vi "一体站流程自动启动.vi"(11 "参数":T1) -> ()   [LabVIEW 2016, in "PLC.lvlib"]
uses:
  PLC.lvlib
  <vilib>/ptbypt/NI_PtbyPt.lvlib
panel:
  out "s? t:f":enum16{"初始化", "采配水启动", "仪器操作", "反冲洗", "结束"}(ring)
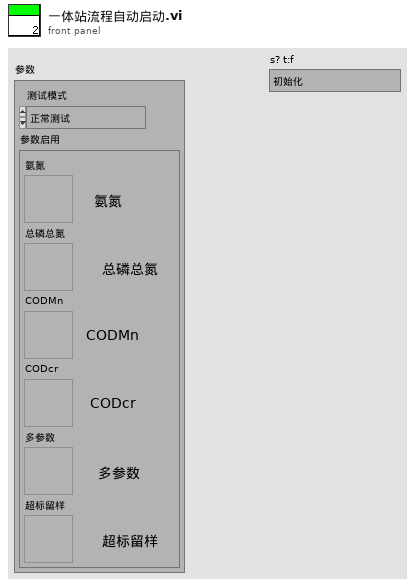
[diagram p1: front panel]
types:
  T1 = cluster{"测试模式":enum16{"正常测试", "集成干预"}, "参数启用":cluster{"氨氮":bool, "总磷总氮":bool, "CODMn":bool, "CODcr":bool, "多参数":bool, "超标留样":bool}}
  T2 = cluster{"命令":string, cluster{"starting address":u16, "holding register value":u16}}
  T3 = enum16{"启动测量", "标样核查", "零点核查", "跨度核查", "空白测试", "平行样测试", "加标回收", "空白校准", "标样校准", "初始化（清洗）", "停止测试", "仪器重启", "校时", "模式设置", "测量间隔设置"}
  T4 = cluster{"时间标识":timestamp, "设备":string, "日志信息":string, "流程参数":string}
  T5 = cluster{"测量模式":enum16{"水样测量", "标样核查", "零点核查", "跨度核查", "空白测试", "加标回收", "平行样", "校零", "校标"}}
  T6 = cluster{"时间标识":timestamp, "设备":string, "日志信息":string}
  T7 = enum16{"空闲", "水样测试", "标样核查", "零点核查", "跨度核查", "空白测试", "平行样测试", "加标回收", "空白校准", "标样校准", "初始化（清洗）"}
  T8 = enum32{"Bad", "Idle", "Run top level", "Running"}
  T9 = cluster{"R0":i16, "R1":i16, "R2":i16, "R3":i16, "R4":i16, "R5":i16, "R6":i16, "R7":i16, "R8":i16, "R9":i16, "R10":i16, "R11":i16, "R12":i16, "R13":i16, "R14":i16, "R15":i16, "R16":i16, "R17":i16, "R18":i16, "R19":i16, "R20":i16, "R21":i16, "R22":i16, "R23":i16, "R24":i16, "R25":i16, "R26":i16, "R27":i16, "R28":i16, "R29":i16, "R30":i16, "R31":i16, "R32":i16, "R33":i16, "R34":i16, "R35":i16, "R36":i16, "R37":i16, "R38":i16, "R39":i16, "R40":i16, "R41":i16, "R42":i16, "R43":i16, "R44":i16, "R45":i16, "R46":i16, "R47":i16, "R48":i16, "R49":i16, "R50":i16, "R51":i16, "R52":i16, "R53":i16, "R54":i16, "R55":i16, "R56":i16}
  T10 = cluster{"R100":i16, "R101":i16, "R102":i16, "R103":i16, "R104":i16, "R105":i16, "R106":i16, "R107":i16, "R108":i16, "R109":i16, "R110":i16, "R111":i16, "R112":i16, "R113":i16, "R114":i16, "R115":i16, "R116":i16, "R117":i16, "R118":i16, "R119":i16, "R120":i16, "R121":i16, "R122":i16, "R123":i16, "R124":i16}
  T11 = cluster{"氨氮":bool, "总磷总氮":bool, "CODmn":bool, "CODCr":bool, "多参数":bool, "超标留样":bool}
  T12 = cluster{"因子编码":u32, "单位":u16, "标样参考值":sgl, "水样数据时间":timestamp, "水样实测值":sgl, "水样数据标识":string, "标样数据时间":timestamp, "标样实测值":sgl, "标样数据标识":string, "空白数据时间":timestamp, "空白实测值":sgl, "空白数据标识":string, "零点核查数据时间":timestamp, "零点核查实测值":sgl, "零点核查数据标识":string, "跨度核查数据时间":timestamp, "跨度核查实测值":sgl, "跨度核查数据标识":string, "加标回收数据时间":timestamp, "加标回收实测值":sgl, "加标回收数据标识":string, "平行样数据时间":timestamp, "平行样实测值":sgl, "平行样数据标识":string, "F0":sgl, "F1":sgl, "F2":sgl, "F3":sgl, "F4":sgl, "F5":sgl, "F6":sgl, "F7":sgl, "温度":sgl, "湿度":sgl, "X值":sgl, "fidrange":u16}
  T13 = cluster{"COD浓度（mg/L)":dbl, "水样启动时间":timestamp, "加标回收启动时间":timestamp, "CODMn工作状态":enum16{"空闲", "水样测试", "标样核查", "零点核查", "跨度核查", "空白测试", "平行样测试", "加标回收", "空白校准", "标样校准", "初始化（清洗）"}, "多列列表框":i32}
  T14 = cluster{"因子编码":u32, "单位":u16, "标样参考值":sgl, "水样数据时间":timestamp, "水样实测值":sgl, "水样数据标识":string, "标样数据时间":timestamp, "标样实测值":sgl, "标样数据标识":string, "空白数据时间":timestamp, "空白实测值":sgl, "空白数据标识":string, "零点核查数据时间":timestamp, "零点核查实测值":sgl, "零点核查数据标识":string, "跨度核查数据时间":timestamp, "跨度核查实测值":sgl, "跨度核查数据标识":string, "加标回收数据时间":timestamp, "加标回收实测值":sgl, "加标回收数据标识":string, "平行样数据时间":timestamp, "平行样实测值":sgl, "平行样数据标识":string}
  T15 = cluster{"氨氮":bool, "总磷总氮":bool, "CODMn":bool, "CODcr":bool, "多参数":bool, "超标留样":bool}
  T16 = cluster{"时间标识":timestamp, "参数":string, "数据类型":string, "集成干预测试浓度值":dbl, "集成干预前测试时间":timestamp, "集成干预前测试浓度值":dbl}
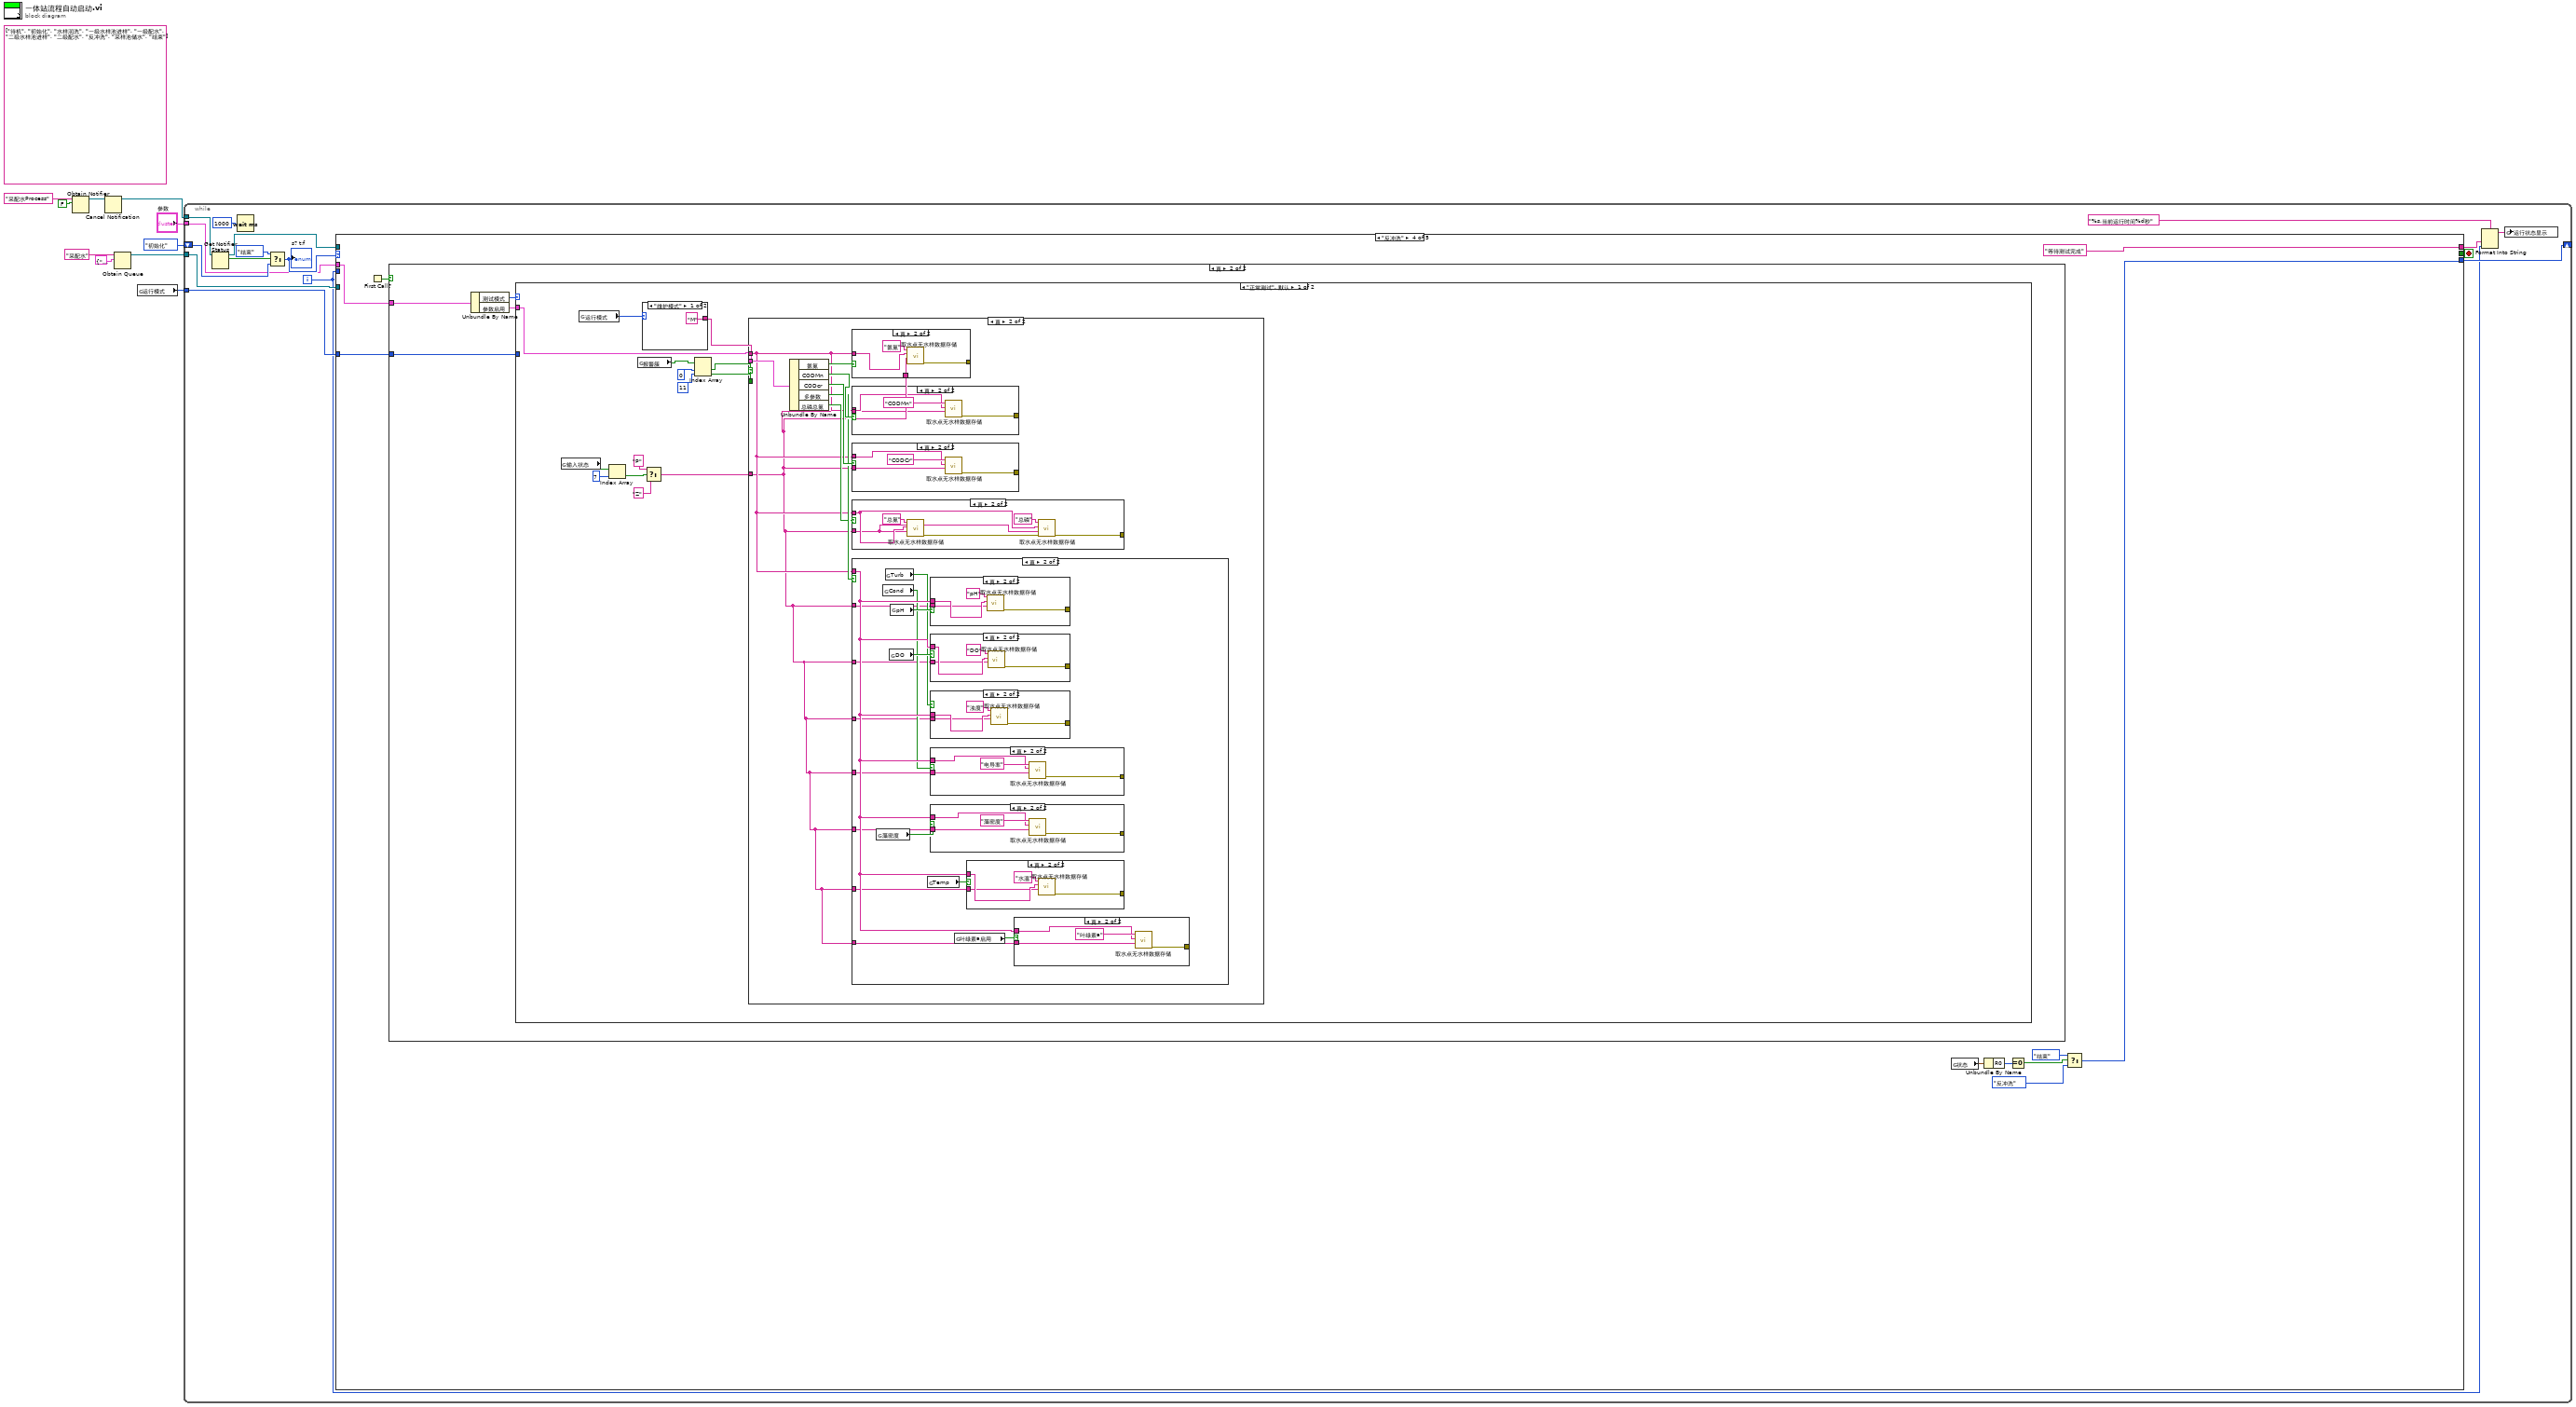
[diagram p0: block diagram]
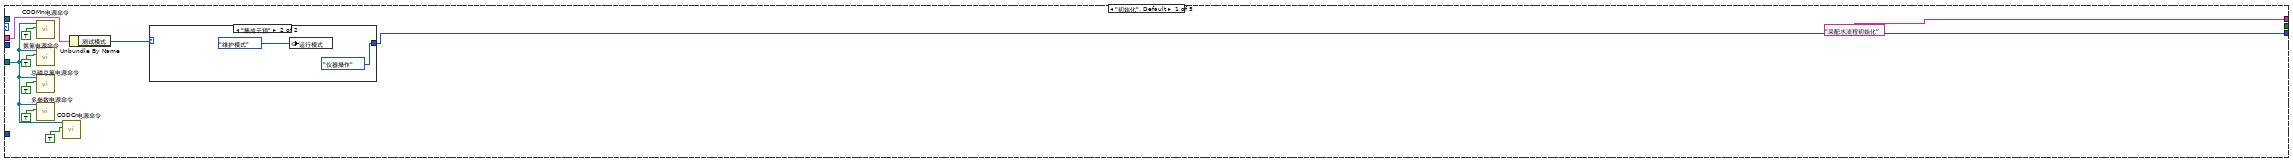
[diagram p2: hidden frame]
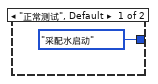
[diagram p3: hidden frame]
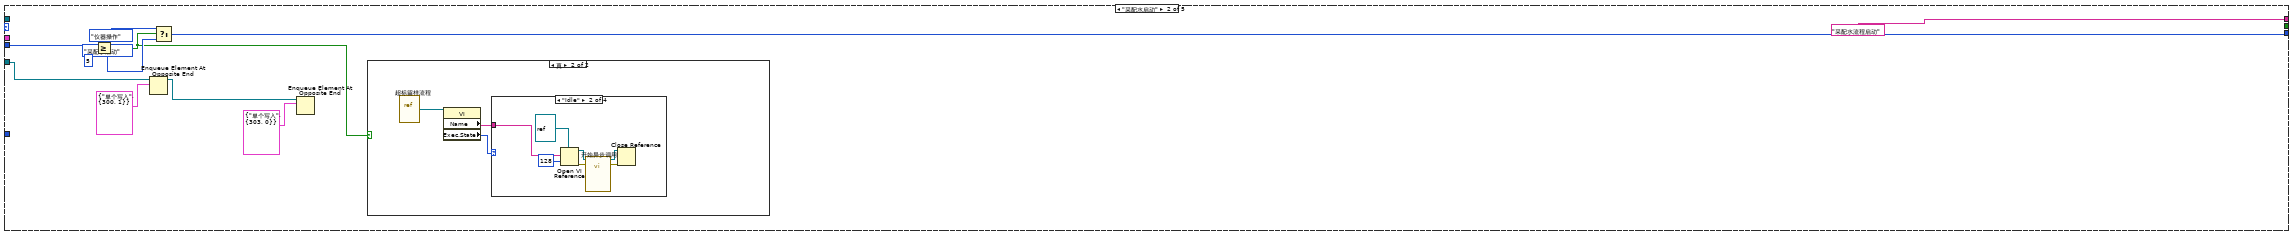
[diagram p4: hidden frame]
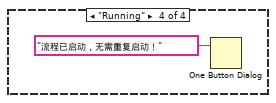
[diagram p8: hidden frame]
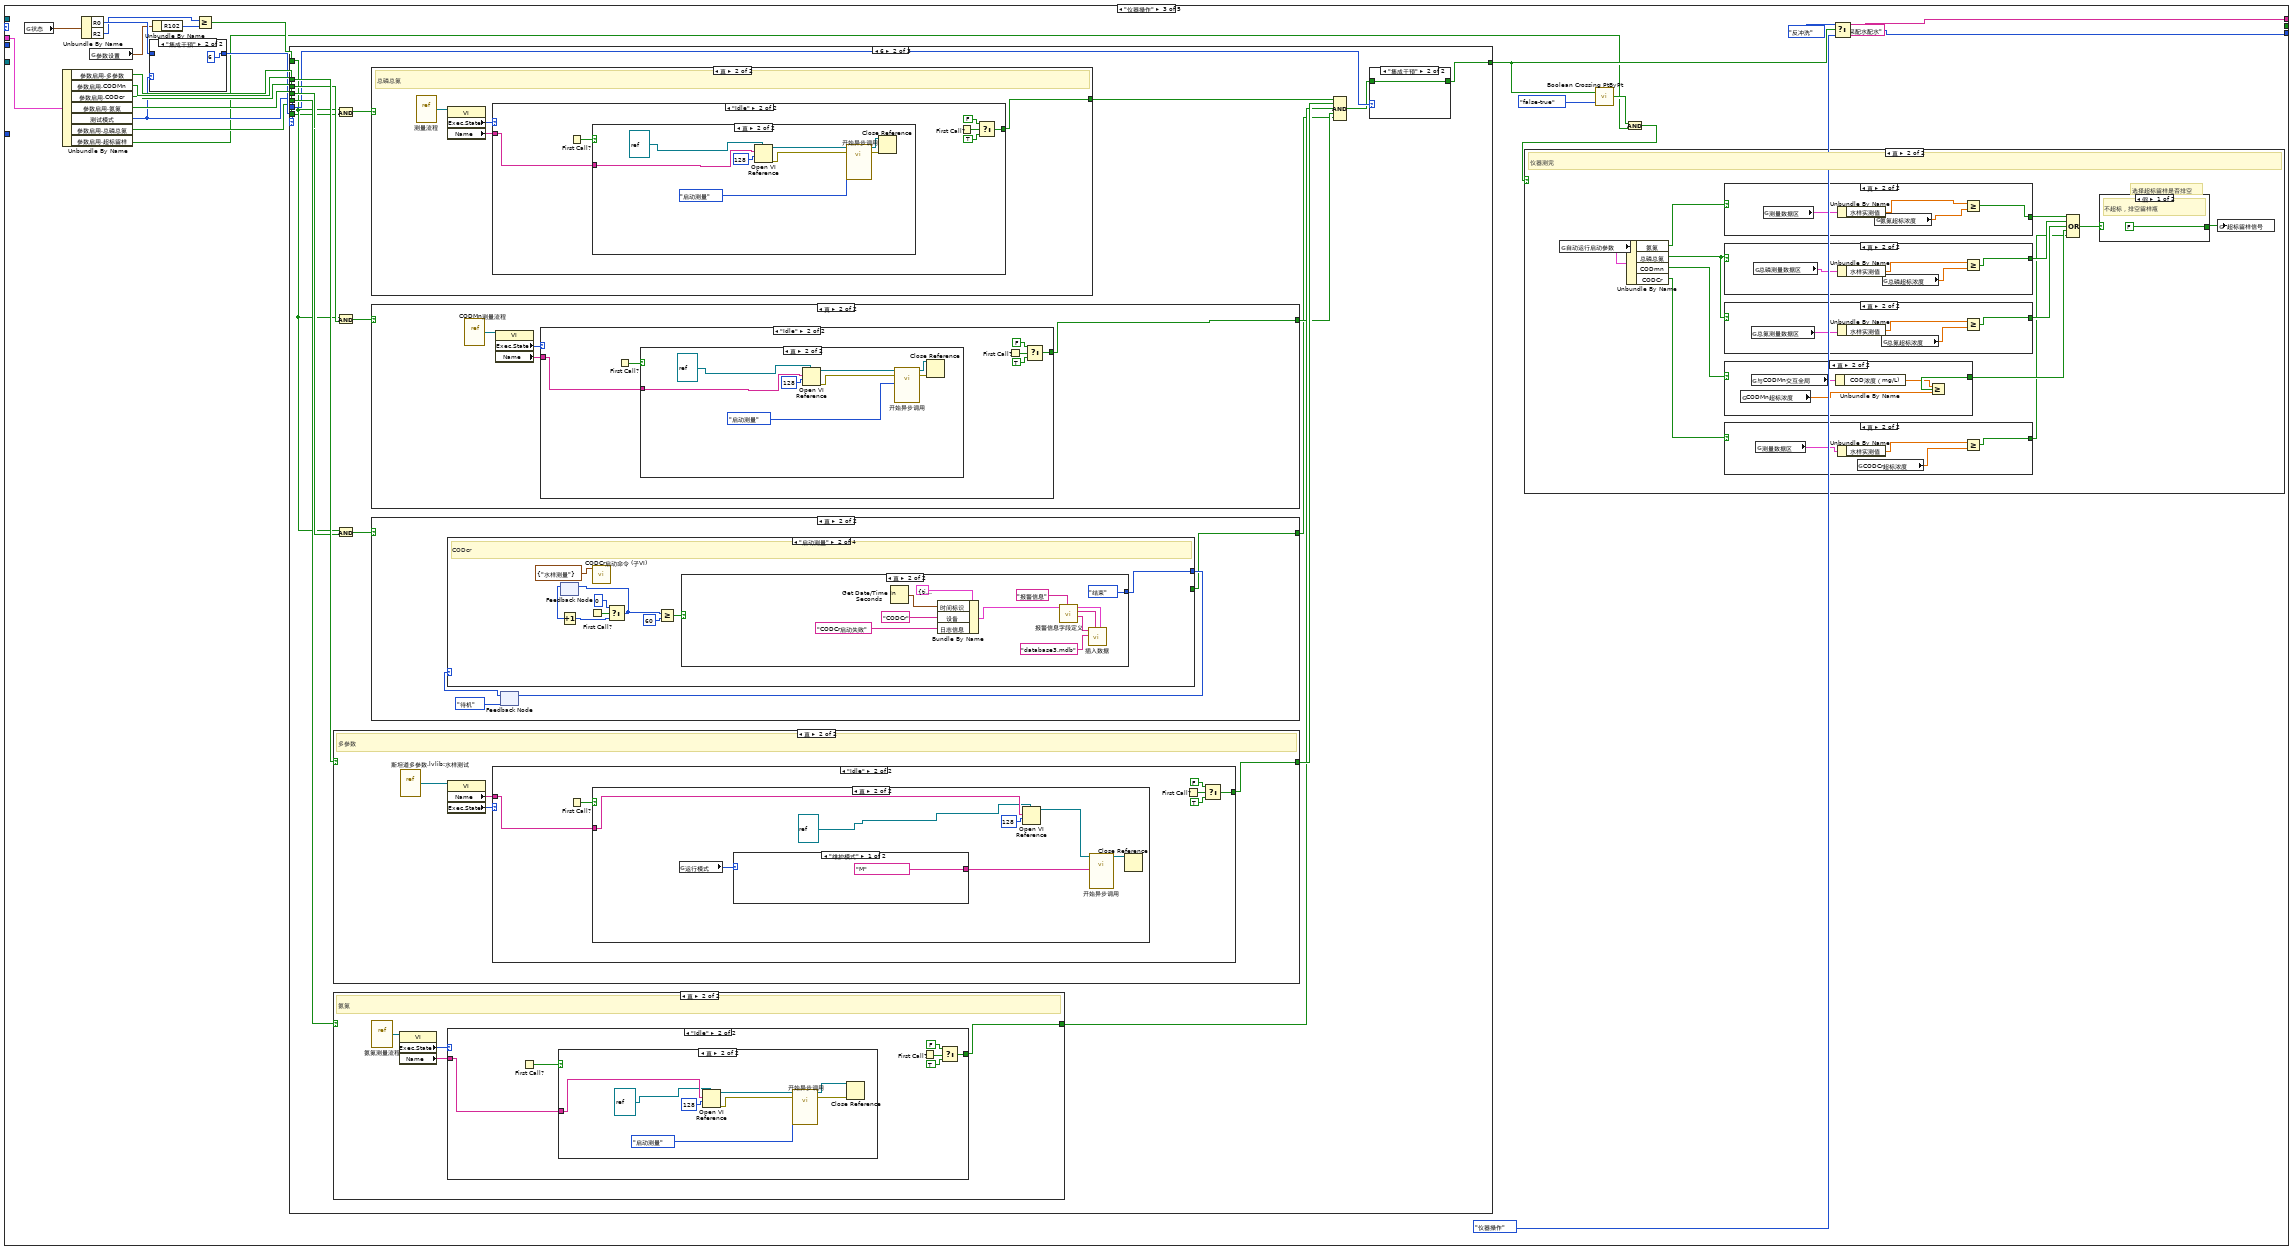
[diagram p9: hidden frame]
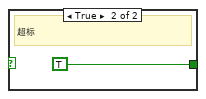
[diagram p11: hidden frame]
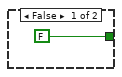
[diagram p12: hidden frame]
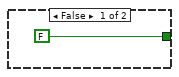
[diagram p13: hidden frame]
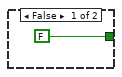
[diagram p14: hidden frame]
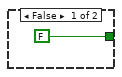
[diagram p15: hidden frame]
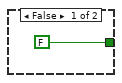
[diagram p16: hidden frame]
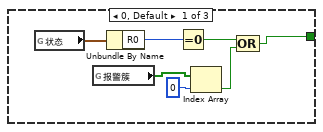
[diagram p18: hidden frame]
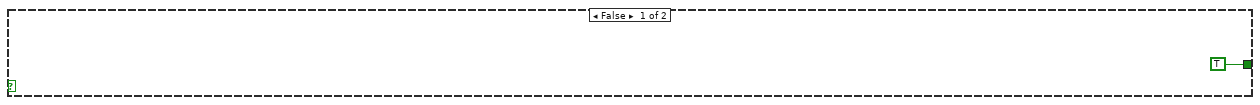
[diagram p19: hidden frame]
diagram:
  (unwired) string[][] [["待机"], ["初始化"], ["水样润洗"], ["一级水样池进样"], ["一级配水"], ["二级水样池进样"], ["二级配水"], ["反冲洗"], ["采样池储水"], ["结束"]] ("项名")
  n1 = Obtain Notifier(name (unnamed)="采配水Process" ("名称（未命名）"), notification data type=FALSE) -> (notifier out=w4:refnum<notifier>)  [unwired: 2 in, 2 out]
  n2 = Cancel Notification(0:w4) -> (8:w3:refnum<notifier>)  [unwired: 1 in, 2 out]
  n3 = Obtain Queue(name (unnamed)="采配水" ("名称（未命名）"), element data type=cluster{"命令":string, "数据":variant} {"命令"="", "数据"=variant}) -> (queue out=w7:refnum<queue>)  [unwired: 3 in, 2 out]
  n4 = global read "系统设置全局变量.vi" "运行模式"() -> (w1:enum16{"维护模式", "常规模式", "应急模式", "质控模式"})
  n5 = while {
    shift-right: [w23] -> _
    shift-left: enum16{"初始化", "采配水启动", "仪器操作", "反冲洗", "结束"}."初始化" ("枚举") -> [w19]
    tunnel: w7 -> [w26]
    tunnel: w3 -> [w22]
    tunnel: "参数" -> [w13]
    tunnel: w1 -> [w12]
    i -> [w11]
    stop <- w25 stop-if-true
    n6 = Get Notifier Status(notifier=w22) -> (notifier out=w14:refnum<notifier>, current notification=w21:bool)  [unwired: 1 in, 3 out]
    n7 = Wait (ms)(milliseconds to wait=u32 1000 ("等待时间（毫秒）")) -> ()  [unwired: 1 out]
    n8 = Select(t=enum16{"初始化", "采配水启动", "仪器操作", "反冲洗", "结束"}."结束" ("枚举"), s=w21, f=w19) -> (s? t:f=w18:enum16{"初始化", "采配水启动", "仪器操作", "反冲洗", "结束"})
    "s? t:f" <- w18
    n9 = case shown="\"反冲洗\"" w18 {
      tunnel: w26 -> [w31 w50 _ _ w476]
      tunnel: [_ _ _ _ TRUE] -> w25
      tunnel: [w30 w43 w80 w285 enum16{"初始化", "采配水启动", "仪器操作", "反冲洗", "结束"}."结束" ("枚举")] -> w23
      tunnel: ["采配水流程初始化" "采配水流程启动" "采配水配水" "等待测试完成" "采配水结束"] -> w15
      tunnel: w14 -> [_ _ _ _ w477]
      tunnel: w13 -> [w28 _ w82 w284 w473]
      tunnel: w12 -> [_ _ _ w281 w472]
      tunnel: w11 -> [_ w48 _ _ _]
      frame "初始化", Default {
        n10 = call "CODMn电源命令.vi"("通电/断电"=TRUE, "队列"=w31) -> ()  [unwired: 9 in, 1 out]
        n11 = call "氨氮电源命令.vi"("通电/断电"=TRUE, "队列"=w31) -> ()  [unwired: 9 in, 1 out]
        n12 = call "总磷总氮电源命令.vi"("通电/断电"=TRUE, "队列"=w31) -> ()  [unwired: 9 in, 1 out]
        n13 = call "多参数电源命令.vi"("通电/断电"=TRUE, "队列"=w31) -> ()  [unwired: 9 in, 1 out]
        n14 = call "CODCr电源命令.vi"("通电/断电"=TRUE, "队列"=w31) -> ()  [unwired: 9 in, 1 out]
        n15 = Unbundle By Name(w28) -> ("测试模式"=w27:enum16{"正常测试", "集成干预"})
        n16 = case shown="\"集成干预\"" w27 {
          tunnel: [enum16{"初始化", "采配水启动", "仪器操作", "反冲洗", "结束"}."采配水启动" ("枚举") enum16{"初始化", "采配水启动", "仪器操作", "反冲洗", "结束"}."仪器操作" ("枚举")] -> w30
          frame "正常测试", Default {
          }
          frame "集成干预" {
            n17 = global write "系统设置全局变量.vi" "运行模式"(enum16{"维护模式", "常规模式", "应急模式", "质控模式"}."维护模式" ("运行模式")) -> ()
          }
        }
      }
      frame "采配水启动" {
        n18 = Greater Or Equal?(x=w48, y=5) -> (x >= y?=w40:bool)
        n19 = Enqueue Element At Opposite End(queue=w50, element=T2 {"命令"="单个写入", {"starting address"=300, "holding register value"=1}} ("元素")) -> (queue out=w41:refnum<queue>)  [unwired: 2 in, 2 out]
        n20 = Select(t=enum16{"初始化", "采配水启动", "仪器操作", "反冲洗", "结束"}."仪器操作" ("枚举"), s=w40, f=enum16{"初始化", "采配水启动", "仪器操作", "反冲洗", "结束"}."采配水启动" ("枚举")) -> (s? t:f=w43:enum16{"初始化", "采配水启动", "仪器操作", "反冲洗", "结束"})
        n21 = Enqueue Element At Opposite End(queue=w41, element=T2 {"命令"="单个写入", {"starting address"=303, "holding register value"=0}} ("元素")) -> ()  [unwired: 2 in, 3 out]
        n22 = case shown="真" w40 {
          frame False {
          }
          frame True {
            n23 = vi-ref "超标留样流程.vi"() -> (w53:refnum<vi>)
            n24 = property class="VI"(reference=w53) -> ("Name"=w52:string, "Exec.State"=w51:T8)  [unwired: 1 in, 2 out]
            n25 = case shown="\"Idle\"" w51 {
              tunnel: w52 -> [_ w56 _ _]
              frame "Bad", Default {
              }
              frame "Idle" {
                n26 = Open VI Reference(type specifier VI Refnum (for type only)=refnum<vi> refnum ("类型说明符VI引用句柄（仅用于类型）"), vi path=w56, options=128 ("选项")) -> (vi reference=w60:refnum<vi>, error out=w55:errorcluster)  [unwired: 3 in]
                n27 = call-by-ref "开始异步调用"(reference=w60, error in=w55) -> (reference out=w59:refnum<vi>, error out=w54:errorcluster)  [unwired: 12 in]
                n28 = Close Reference(reference=w59, error in (no error)=w54) -> ()  [unwired: 1 out]
              }
              frame "Run top level" {
              }
              frame "Running" {
                n29 = One Button Dialog(message="流程已启动，无需重复启动！" ("消息")) -> ()  [unwired: 1 in, 1 out]
              }
            }
          }
        }
      }
      frame "仪器操作" {
        n30 = global read "采配水全局变量.vi" "状态"() -> (w84:T9)
        n31 = Unbundle By Name(w82) -> ("参数启用.多参数"=w78:bool, "参数启用.CODMn"=w77:bool, "参数启用.CODcr"=w76:bool, "参数启用.氨氮"=w75:bool, "测试模式"=w68:enum16{"正常测试", "集成干预"}, "参数启用.总磷总氮"=w67:bool, "参数启用.超标留样"=w62:bool)
        n32 = Unbundle By Name(w84) -> ("R0"=w74:i16, "R2"=w69:i16)
        n33 = global read "采配水全局变量.vi" "参数设置"() -> (w71:T10)
        n34 = case shown="\"集成干预\"" w68 {
          tunnel: w74 -> [w124 _]
          tunnel: [w124 i16 6 ("R0")] -> w73
          frame "正常测试", Default {
          }
          frame "集成干预" {
          }
        }
        n35 = Unbundle By Name(w71) -> ("R102"=w72:i16)
        n36 = Greater Or Equal?(x=w69, y=w72) -> (x >= y?=w70:bool)
        n37 = case shown="6" w73 {
          tunnel: [w127 w137 TRUE] -> w63
          tunnel: w78 -> [_ w149 _]
          tunnel: w77 -> [_ w148 _]
          tunnel: w76 -> [_ w145 _]
          tunnel: w75 -> [_ w144 _]
          tunnel: w70 -> [_ w136 _]
          tunnel: w68 -> [_ w139 _]
          tunnel: w67 -> [_ w135 _]
          frame 0, Default {
            n38 = global read "采配水全局变量.vi" "状态"() -> (w130:T9)
            n39 = global read "采配水全局变量.vi" "报警簇"() -> (w131:bool[])
            n40 = Unbundle By Name(w130) -> ("R0"=w129:i16)
            n41 = Equal To 0?(x=w129) -> (x = 0?=w132:bool)
            n42 = Index Array(array=w131, index=0 ("索引")) -> (element=w126:bool)
            n43 = Compound Arithmetic op=OR ("复合运算")(w132, w126) -> (w127:bool)
          }
          frame 6 {
            n44 = case shown="真" w149 {
              tunnel: [TRUE ("t") w261] -> w143
              frame False {
              }
              frame True {
                # "多参数"
                n45 = vi-ref "斯坦道多参数.lvlib:水样测试.vi"() -> (w263:refnum<vi>)
                n46 = property class="VI"(reference=w263) -> ("Name"=w262:string, "Exec.State"=w264:T8)  [unwired: 1 in, 2 out]
                n47 = case shown="\"Idle\"" w264 {
                  tunnel: w262 -> [_ w270]
                  tunnel: [_ w265] -> w261
                  frame "Bad", Default {
                  }
                  frame "Idle" {
                    n48 = First Call?() -> (First Call?: T/F=w269:bool)
                    n49 = case shown="真" w269 {
                      tunnel: w270 -> [_ w276]
                      frame False {
                      }
                      frame True {
                        n50 = global read "系统设置全局变量.vi" "运行模式"() -> (w273:enum16{"维护模式", "常规模式", "应急模式", "质控模式"})
                        n51 = case shown="\"维护模式\"" w273 {
                          tunnel: ["M" ("数据标记表") "N" ("数据标记表")] -> w272
                          frame "维护模式" {
                          }
                          frame "常规模式", Default {
                          }
                        }
                        n52 = Open VI Reference(type specifier VI Refnum (for type only)=refnum<vi> refnum, vi path=w276, options=128 ("选项")) -> (vi reference=w275:refnum<vi>)  [unwired: 3 in, 1 out]
                        n53 = call-by-ref "开始异步调用"(reference=w275, "数据标记表"=w272) -> (reference out=w274:refnum<vi>)  [unwired: 12 in, 1 out]
                        n54 = Close Reference(reference=w274) -> ()  [unwired: 1 in, 1 out]
                      }
                    }
                    n55 = First Call?() -> (First Call?: T/F=w268:bool)
                    n56 = Select(t=FALSE, s=w268, f=TRUE) -> (s? t:f=w265:bool)
                  }
                }
              }
            }
            n57 = case "条件结构" shown="真" w144 {
              tunnel: [TRUE ("t") w171] -> w142
              frame False {
              }
              frame True {
                # "氨氮"
                n58 = vi-ref "氨氮测量流程.vi"() -> (w174:refnum<vi>)
                n59 = property class="VI"(reference=w174) -> ("Exec.State"=w173:T8, "Name"=w172:string)  [unwired: 1 in, 2 out]
                n60 = case shown="\"Idle\"" w173 {
                  tunnel: w172 -> [_ w180]
                  tunnel: [_ w175] -> w171
                  frame "Bad", Default {
                  }
                  frame "Idle" {
                    n61 = First Call?() -> (First Call?: T/F=w179:bool)
                    n62 = case shown="真" w179 {
                      tunnel: w180 -> [_ w185]
                      frame False {
                      }
                      frame True {
                        n63 = Open VI Reference(type specifier VI Refnum (for type only)=refnum<vi> refnum, vi path=w185, options=128 ("选项")) -> (vi reference=w183:refnum<vi>, error out=w186:errorcluster)  [unwired: 3 in]
                        n64 = call-by-ref "开始异步调用"(reference=w183, error in=w186, "控制命令"=T3."启动测量") -> (reference out=w187:refnum<vi>, error out=w188:errorcluster)  [unwired: 11 in]
                        n65 = Close Reference(reference=w187, error in (no error)=w188) -> ()  [unwired: 1 out]
                      }
                    }
                    n66 = First Call?() -> (First Call?: T/F=w178:bool)
                    n67 = Select(t=FALSE, s=w178, f=TRUE) -> (s? t:f=w175:bool)
                  }
                }
              }
            }
            n68 = And(x=w136, y=w135) -> (x .and. y?=w134:bool)
            n69 = And(x=w136, y=w148) -> (x .and. y?=w147:bool)
            n70 = And(x=w136, y=w145) -> (x .and. y?=w146:bool)
            n71 = case "条件结构" shown="真" w134 {
              tunnel: [TRUE ("t") w151] -> w133
              frame False {
              }
              frame True {
                # "总磷总氮"
                n72 = vi-ref "测量流程.vi"() -> (w154:refnum<vi>)
                n73 = property class="VI"(reference=w154) -> ("Exec.State"=w153:T8, "Name"=w152:string)  [unwired: 1 in, 2 out]
                n74 = case shown="\"Idle\"" w153 {
                  tunnel: w152 -> [_ w160]
                  tunnel: [_ w155] -> w151
                  frame "Bad", Default {
                  }
                  frame "Idle" {
                    n75 = First Call?() -> (First Call?: T/F=w159:bool)
                    n76 = case shown="真" w159 {
                      tunnel: w160 -> [_ w165]
                      frame False {
                      }
                      frame True {
                        n77 = Open VI Reference(type specifier VI Refnum (for type only)=refnum<vi> refnum, vi path=w165, options=128 ("选项")) -> (vi reference=w163:refnum<vi>, error out=w166:errorcluster)  [unwired: 3 in]
                        n78 = call-by-ref "开始异步调用"(reference=w163, error in=w166, "控制命令"=T3."启动测量") -> (reference out=w167:refnum<vi>, error out=w168:errorcluster)  [unwired: 11 in]
                        n79 = Close Reference(reference=w167, error in (no error)=w168) -> ()  [unwired: 1 out]
                      }
                    }
                    n80 = First Call?() -> (First Call?: T/F=w158:bool)
                    n81 = Select(t=FALSE, s=w158, f=TRUE) -> (s? t:f=w155:bool)
                  }
                }
              }
            }
            n82 = case shown="真" w147 {
              tunnel: [TRUE w242] -> w141
              frame False {
              }
              frame True {
                n83 = vi-ref "CODMn测量流程.vi"() -> (w243:refnum<vi>)
                n84 = property class="VI"(reference=w243) -> ("Exec.State"=w244:T8, "Name"=w245:string)  [unwired: 1 in, 2 out]
                n85 = case shown="\"Idle\"" w244 {
                  tunnel: w245 -> [_ w251]
                  tunnel: [_ w246] -> w242
                  frame "Bad", Default {
                  }
                  frame "Idle" {
                    n86 = First Call?() -> (First Call?: T/F=w250:bool)
                    n87 = case shown="真" w250 {
                      tunnel: w251 -> [_ w256]
                      frame False {
                      }
                      frame True {
                        n88 = Open VI Reference(type specifier VI Refnum (for type only)=refnum<vi> refnum, vi path=w256, options=128 ("选项")) -> (vi reference=w254:refnum<vi>, error out=w257:errorcluster)  [unwired: 3 in]
                        n89 = call-by-ref "开始异步调用"(reference=w254, error in=w257, "控制命令"=T3."启动测量") -> (reference out=w258:refnum<vi>, error out=w259:errorcluster)  [unwired: 11 in]
                        n90 = Close Reference(reference=w258, error in (no error)=w259) -> ()  [unwired: 1 out]
                      }
                    }
                    n91 = First Call?() -> (First Call?: T/F=w249:bool)
                    n92 = Select(t=FALSE, s=w249, f=TRUE) -> (s? t:f=w246:bool)
                  }
                }
              }
            }
            n93 = case shown="真" w146 {
              tunnel: [TRUE w190] -> w140
              frame False {
              }
              frame True {
                n94 = feedback #1(enum16{"待机", "启动测量", "测量中", "结束"}."待机") -> (w192:enum16{"待机", "启动测量", "测量中", "结束"})
                n95 = case shown="\"启动测量\"" w192 {
                  tunnel: [enum16{"待机", "启动测量", "测量中", "结束"}."启动测量" w208 w228 enum16{"待机", "启动测量", "测量中", "结束"}."结束"] -> w191
                  tunnel: [_ _ _ TRUE] -> w190
                  frame "待机", Default {
                    n96 = Get Date/Time In Seconds() -> (seconds since 1Jan1904=w198:timestamp)
                    n97 = Bundle By Name(cluster=T4 {"时间标识"=timestamp(0 s since 1904-01-01), "设备"="", "日志信息"="", "流程参数"=""} ("data in"), "时间标识"=w198, "设备"="CODCr", "日志信息"="-->>CODCr启动") -> (w194:T4)
                    n98 = call "总磷总氮操作日志.vi"("data in"=w194) -> ()  [unwired: 11 in]
                  }
                  frame "启动测量" {
                    # "CODcr"
                    n99 = feedback #2() -> (w204:i32)  [unwired: 1 in]
                    n100 = Increment(x=w204) -> (x+1=w205:i32)
                    n101 = First Call?() -> (First Call?: T/F=w203:bool)
                    n102 = call "CODCr启动命令 (子VI).vi"("启动测量模式"=T5 {"测量模式"=enum."水样测量"}) -> ()  [unwired: 11 in]
                    n103 = Select(t=0, s=w203, f=w205) -> (s? t:f=w206:i32)
                    n104 = feedback-in #2(w206) -> ()
                    n105 = Greater Or Equal?(x=w206, y=60) -> (x >= y?=w201:bool)
                    n106 = case shown="真" w201 {
                      tunnel: [w209 enum16{"待机", "启动测量", "测量中", "结束"}."结束"] -> w208
                      frame False {
                        n107 = global read "CODcr全局变量.vi" "工作状态"() -> (w210:T7)
                        n108 = Not Equal To 0?(x=w210) -> (x != 0?=w211:bool)
                        n109 = Select(t=enum16{"待机", "启动测量", "测量中", "结束"}."测量中", s=w211, f=enum16{"待机", "启动测量", "测量中", "结束"}."启动测量") -> (s? t:f=w209:enum16{"待机", "启动测量", "测量中", "结束"})
                      }
                      frame True {
                        n110 = Get Date/Time In Seconds() -> (seconds since 1Jan1904=w220:timestamp)
                        n111 = Bundle By Name(cluster=T6 {"时间标识"=timestamp(0 s since 1904-01-01), "设备"="", "日志信息"=""} ("data in"), "时间标识"=w220, "设备"="CODCr", "日志信息"="CODCr启动失败") -> (w214:T6)
                        n112 = call "报警信息字段定义.vi"("table输入"="报警信息", "data in"=w214) -> ("table输出"=w217:string, "columns"=w218:string[], "data out"=w219:T6)  [unwired: 7 in]
                        n113 = call "插入数据.vi"("data"=w219, "columns"=w218, "database"="database3.mdb", "table"=w217) -> ()  [unwired: 7 in, 1 out]
                      }
                    }
                  }
                  frame "测量中" {
                    n114 = global read "CODcr全局变量.vi" "工作状态"() -> (w227:T7)
                    n115 = Equal?(x=w227, y=T7."空闲" ("工作状态")) -> (x = y?=w226:bool)
                    n116 = case shown="假" w226 {
                      tunnel: [w229 enum16{"待机", "启动测量", "测量中", "结束"}."结束"] -> w228
                      frame False {
                        n117 = flat-sequence {
                          tunnel: [enum16{"待机", "启动测量", "测量中", "结束"}."测量中"] -> w229
                          frame #0 {
                            n118 = Wait (ms)(milliseconds to wait=u32 1000 ("等待时间（毫秒）")) -> ()  [unwired: 1 out]
                          }
                          frame #1 {
                          }
                        }
                      }
                      frame True {
                      }
                    }
                  }
                  frame "结束" {
                    n119 = First Call?() -> (First Call?: T/F=w233:bool)
                    n120 = case shown="真" w233 {
                      frame False {
                      }
                      frame True {
                        n121 = Get Date/Time In Seconds() -> (seconds since 1Jan1904=w240:timestamp)
                        n122 = Bundle By Name(cluster=T4 {"时间标识"=timestamp(0 s since 1904-01-01), "设备"="", "日志信息"="", "流程参数"=""} ("data in"), "时间标识"=w240, "设备"="CODCr", "日志信息"="-->>CODCr停止") -> (w236:T4)
                        n123 = call "总磷总氮操作日志.vi"("data in"=w236) -> ()  [unwired: 11 in]
                      }
                    }
                  }
                }
                n124 = feedback-in #1(w191) -> ()
              }
            }
            n125 = Compound Arithmetic op=AND ("复合运算")(w133, w143, w142, w141, w140) -> (w138:bool)
            n126 = case shown="\"集成干预\"" w139 {
              tunnel: w138 -> [_ w169]
              tunnel: [_ w169] -> w137
              frame "正常测试", Default {
              }
              frame "集成干预" {
              }
            }
          }
          frame 7..9 {
          }
        }
        n127 = call <vilib>:"Boolean Crossing PtByPt.vi"("direction"=enum16{"either", "false-true", "true-false"}."false-true", "input"=w63) -> ("crossing"=w65:bool)  [unwired: 1 in]
        n128 = And(x=w65, y=w62) -> (x .and. y?=w64:bool)
        n129 = case shown="真" w64 {
          frame False {
          }
          frame True {
            # "选择超标留样是否排空"
            # "仪器测完"
            n130 = global read "系统设置全局变量.vi" "自动运行启动参数"() -> (w89:T11)
            n131 = Unbundle By Name(w89) -> ("氨氮"=w88:bool, "总磷总氮"=w87:bool, "CODmn"=w86:bool, "CODCr"=w85:bool)
            n132 = case shown="真" w88 {
              tunnel: [FALSE w122] -> w96
              frame False {
              }
              frame True {
                n133 = global read "VAR氨氮全局变量.vi" "测量数据区"() -> (w121:T12)
                n134 = Unbundle By Name(w121) -> ("水样实测值"=w123:sgl)
                n135 = global read "外部交互全局.vi" "氨氮超标浓度"() -> (w120:dbl)
                n136 = Greater Or Equal?(x=w123, y=w120) -> (x >= y?=w122:bool)
              }
            }
            n137 = case shown="真" w87 {
              tunnel: [FALSE w118] -> w95
              frame False {
              }
              frame True {
                n138 = global read "VAR总磷总氮全局变量.vi" "总磷测量数据区"() -> (w115:T12)
                n139 = Unbundle By Name(w115) -> ("水样实测值"=w117:sgl)
                n140 = global read "外部交互全局.vi" "总磷超标浓度"() -> (w116:dbl)
                n141 = Greater Or Equal?(x=w117, y=w116) -> (x >= y?=w118:bool)
              }
            }
            n142 = case shown="真" w87 {
              tunnel: [FALSE w113] -> w94
              frame False {
              }
              frame True {
                n143 = global read "VAR总磷总氮全局变量.vi" "总氮测量数据区"() -> (w110:T12)
                n144 = Unbundle By Name(w110) -> ("水样实测值"=w112:sgl)
                n145 = global read "外部交互全局.vi" "总氮超标浓度"() -> (w111:dbl)
                n146 = Greater Or Equal?(x=w112, y=w111) -> (x >= y?=w113:bool)
              }
            }
            n147 = case shown="真" w86 {
              tunnel: [FALSE w108] -> w93
              frame False {
              }
              frame True {
                n148 = global read "外部交互全局.vi" "CODMn超标浓度"() -> (w107:dbl)
                n149 = global read "modbus slave全局.vi" "与CODMn交互全局"() -> (w106:T13)
                n150 = Unbundle By Name(w106) -> ("COD浓度（mg/L)"=w105:dbl)
                n151 = Greater Or Equal?(x=w105, y=w107) -> (x >= y?=w108:bool)
              }
            }
            n152 = case shown="真" w85 {
              tunnel: [FALSE w103] -> w92
              frame False {
              }
              frame True {
                n153 = global read "CODcr全局变量.vi" "测量数据区"() -> (w100:T14)
                n154 = Unbundle By Name(w100) -> ("水样实测值"=w102:sgl)
                n155 = global read "外部交互全局.vi" "CODCr超标浓度"() -> (w101:dbl)
                n156 = Greater Or Equal?(x=w102, y=w101) -> (x >= y?=w103:bool)
              }
            }
            n157 = Compound Arithmetic op=OR ("复合运算")(w96, w95, w94, w93, w92) -> (w91:bool)
            n158 = case shown="假" w91 {
              tunnel: [FALSE ("超标留样信号") TRUE ("超标留样信号")] -> w90
              frame False {
                # "不超标，排空留样瓶"
              }
              frame True {
                # "超标"
              }
            }
            n159 = global write "外部交互全局.vi" "超标留样信号"(w90) -> ()
          }
        }
        n160 = Select(t=enum16{"初始化", "采配水启动", "仪器操作", "反冲洗", "结束"}."反冲洗" ("枚举"), s=w63, f=enum16{"初始化", "采配水启动", "仪器操作", "反冲洗", "结束"}."仪器操作" ("枚举")) -> (s? t:f=w80:enum16{"初始化", "采配水启动", "仪器操作", "反冲洗", "结束"})
      }
      frame "反冲洗" {
        n161 = First Call?() -> (First Call?: T/F=w282:bool)
        n162 = case shown="真" w282 {
          tunnel: w284 -> [_ w294]
          tunnel: w281 -> [_ w291]
          frame False {
          }
          frame True {
            n163 = Unbundle By Name(w294) -> ("测试模式"=w293:enum16{"正常测试", "集成干预"}, "参数启用"=w292:T15)
            n164 = case shown="\"正常测试\", 默认" w293 {
              tunnel: w292 -> [w303 w396]
              tunnel: w291 -> [_ w390]
              frame "正常测试", Default {
                n165 = global read "采配水全局变量.vi" "输入状态"() -> (w300:bool[])
                n166 = global read "系统设置全局变量.vi" "运行模式"() -> (w301:enum16{"维护模式", "常规模式", "应急模式", "质控模式"})
                n167 = Index Array(array=w300, index=7 ("索引")) -> (element=w298:bool)
                n168 = global read "采配水全局变量.vi" "报警簇"() -> (w308:bool[])
                n169 = case shown="\"维护模式\"" w301 {
                  tunnel: ["M" ("table") "N" ("table")] -> w302
                  frame "维护模式" {
                  }
                  frame "常规模式", Default {
                  }
                }
                n170 = Select(t="P" ("数据标识"), s=w298, f="Z" ("数据标识")) -> (s? t:f=w295:string)
                n171 = Index Array(array=w308, index #1=0 ("索引"), index #2=11 ("索引")) -> (element #1=w305:bool, element #2=w304:bool)
                n172 = case shown="真" w305 {
                  tunnel: w304 -> [w314 _]
                  tunnel: w303 -> [w313 w328]
                  tunnel: w302 -> [w311 w322]
                  tunnel: w295 -> [_ w321]
                  frame False {
                    n173 = Unbundle By Name(w313) -> ("氨氮"=w312:bool)
                    n174 = case shown="真" w314 {
                      tunnel: w312 -> [_ w316]
                      tunnel: w311 -> [_ w315]
                      frame False {
                      }
                      frame True {
                        n175 = case shown="真" w316 {
                          tunnel: w315 -> [_ w317]
                          tunnel: [_ w318] -> _
                          frame False {
                          }
                          frame True {
                            n176 = call "取水点无水样数据存储.vi"("数据标识"="lw", "数据类型"=w317, "table"="氨氮") -> ("error out"=w318:errorcluster)  [unwired: 8 in]
                          }
                        }
                      }
                    }
                  }
                  frame True {
                    n177 = Unbundle By Name(w328) -> ("氨氮"=w327:bool, "CODMn"=w326:bool, "CODcr"=w325:bool, "多参数"=w324:bool, "总磷总氮"=w323:bool)
                    n178 = case shown="真" w327 {
                      tunnel: w322 -> [_ w387]
                      tunnel: [_ w388] -> _
                      tunnel: w321 -> [_ w386]
                      frame False {
                      }
                      frame True {
                        n179 = call "取水点无水样数据存储.vi"("数据标识"=w386, "数据类型"=w387, "table"="氨氮") -> ("error out"=w388:errorcluster)  [unwired: 8 in]
                      }
                    }
                    n180 = case shown="真" w326 {
                      tunnel: w322 -> [_ w384]
                      tunnel: [_ w383] -> _
                      tunnel: w321 -> [_ w382]
                      frame False {
                      }
                      frame True {
                        n181 = call "取水点无水样数据存储.vi"("数据标识"=w382, "数据类型"=w384, "table"="CODMn") -> ("error out"=w383:errorcluster)  [unwired: 8 in]
                      }
                    }
                    n182 = case shown="真" w325 {
                      tunnel: w322 -> [_ w380]
                      tunnel: [_ w379] -> _
                      tunnel: w321 -> [_ w378]
                      frame False {
                      }
                      frame True {
                        n183 = call "取水点无水样数据存储.vi"("数据标识"=w378, "数据类型"=w380, "table"="CODCr") -> ("error out"=w379:errorcluster)  [unwired: 8 in]
                      }
                    }
                    n184 = case shown="真" w323 {
                      tunnel: w322 -> [_ w331]
                      tunnel: [_ w330] -> _
                      tunnel: w321 -> [_ w329]
                      frame False {
                      }
                      frame True {
                        n185 = call "取水点无水样数据存储.vi"("数据标识"=w329, "数据类型"=w331, "table"="总氮") -> ("error out"=w332:errorcluster)  [unwired: 8 in]
                        n186 = call "取水点无水样数据存储.vi"("error in (no error)"=w332, "数据标识"=w329, "数据类型"=w331, "table"="总磷") -> ("error out"=w330:errorcluster)  [unwired: 7 in]
                      }
                    }
                    n187 = case shown="真" w324 {
                      tunnel: w322 -> [_ w349]
                      tunnel: w321 -> [_ w341]
                      tunnel: w321 -> [_ w340]
                      tunnel: w321 -> [_ w339]
                      tunnel: w321 -> [_ w338]
                      tunnel: w321 -> [_ w337]
                      tunnel: w321 -> [_ w336]
                      tunnel: w321 -> [_ w335]
                      frame False {
                      }
                      frame True {
                        n188 = global read "断电保存变量.vi" "藻密度"() -> (w342:bool)
                        n189 = global read "断电保存变量.vi" "Cond"() -> (w344:bool)
                        n190 = global read "断电保存变量.vi" "Turb"() -> (w345:bool)
                        n191 = global read "断电保存变量.vi" "DO"() -> (w346:bool)
                        n192 = global read "断电保存变量.vi" "pH"() -> (w347:bool)
                        n193 = global read "断电保存变量.vi" "Temp"() -> (w348:bool)
                        n194 = case shown="真" w347 {
                          tunnel: w349 -> [_ w372]
                          tunnel: [_ w371] -> _
                          tunnel: w341 -> [_ w370]
                          frame False {
                          }
                          frame True {
                            n195 = call "取水点无水样数据存储.vi"("数据标识"=w370, "数据类型"=w372, "table"="pH") -> ("error out"=w371:errorcluster)  [unwired: 8 in]
                          }
                        }
                        n196 = case shown="真" w346 {
                          tunnel: w349 -> [_ w368]
                          tunnel: [_ w367] -> _
                          tunnel: w340 -> [_ w366]
                          frame False {
                          }
                          frame True {
                            n197 = call "取水点无水样数据存储.vi"("数据标识"=w366, "数据类型"=w368, "table"="DO") -> ("error out"=w367:errorcluster)  [unwired: 8 in]
                          }
                        }
                        n198 = case shown="真" w345 {
                          tunnel: w349 -> [_ w360]
                          tunnel: [_ w359] -> _
                          tunnel: w339 -> [_ w358]
                          frame False {
                          }
                          frame True {
                            n199 = call "取水点无水样数据存储.vi"("数据标识"=w358, "数据类型"=w360, "table"="浊度") -> ("error out"=w359:errorcluster)  [unwired: 8 in]
                          }
                        }
                        n200 = case shown="真" w344 {
                          tunnel: w349 -> [_ w364]
                          tunnel: [_ w363] -> _
                          tunnel: w338 -> [_ w362]
                          frame False {
                          }
                          frame True {
                            n201 = call "取水点无水样数据存储.vi"("数据标识"=w362, "数据类型"=w364, "table"="电导率") -> ("error out"=w363:errorcluster)  [unwired: 8 in]
                          }
                        }
                        n202 = case shown="真" w342 {
                          tunnel: w349 -> [_ w352]
                          tunnel: [_ w351] -> _
                          tunnel: w337 -> [_ w350]
                          frame False {
                          }
                          frame True {
                            n203 = call "取水点无水样数据存储.vi"("数据标识"=w350, "数据类型"=w352, "table"="藻密度") -> ("error out"=w351:errorcluster)  [unwired: 8 in]
                          }
                        }
                        n204 = global read "断电保存变量.vi" "叶绿素a启用"() -> (w343:bool)
                        n205 = case shown="真" w348 {
                          tunnel: w349 -> [_ w376]
                          tunnel: [_ w375] -> _
                          tunnel: w336 -> [_ w374]
                          frame False {
                          }
                          frame True {
                            n206 = call "取水点无水样数据存储.vi"("数据标识"=w374, "数据类型"=w376, "table"="水温") -> ("error out"=w375:errorcluster)  [unwired: 8 in]
                          }
                        }
                        n207 = case shown="真" w343 {
                          tunnel: w349 -> [_ w356]
                          tunnel: [_ w355] -> _
                          tunnel: w335 -> [_ w354]
                          frame False {
                          }
                          frame True {
                            n208 = call "取水点无水样数据存储.vi"("数据标识"=w354, "数据类型"=w356, "table"="叶绿素a") -> ("error out"=w355:errorcluster)  [unwired: 8 in]
                          }
                        }
                      }
                    }
                  }
                }
              }
              frame "集成干预" {
                n209 = Unbundle By Name(w396) -> ("氨氮"=w395:bool, "CODMn"=w394:bool, "CODcr"=w393:bool, "多参数"=w392:bool, "总磷总氮"=w391:bool)
                n210 = case shown="真" w395 {
                  tunnel: w390 -> [_ w468]
                  frame False {
                  }
                  frame True {
                    n211 = call "获取最近两组水样测试数据.vi"("运行模式"=w468, "table"="氨氮") -> ("error out"=w469:errorcluster, "存储变量"=w470:T16)  [unwired: 8 in]
                    n212 = call "集成干预测试数据存储.vi"("error in (no error)"=w469, "存储变量"=w470) -> ()  [unwired: 9 in, 1 out]
                  }
                }
                n213 = case shown="真" w392 {
                  tunnel: w390 -> [_ w405]
                  frame False {
                  }
                  frame True {
                    n214 = global read "断电保存变量.vi" "Temp"() -> (w412:bool)
                    n215 = case shown="真" w412 {
                      tunnel: [_ w456] -> w418
                      tunnel: w405 -> [_ w455]
                      frame False {
                      }
                      frame True {
                        n216 = call "获取最近两组水样测试数据.vi"("运行模式"=w455, "table"="水温") -> ("error out"=w459:errorcluster, "存储变量"=w458:T16)  [unwired: 8 in]
                        n217 = call "集成干预测试数据存储.vi"("error in (no error)"=w459, "存储变量"=w458) -> ("error out"=w456:errorcluster)  [unwired: 9 in]
                      }
                    }
                    n218 = global read "断电保存变量.vi" "pH"() -> (w411:bool)
                    n219 = case shown="真" w411 {
                      tunnel: [_ w451] -> w417
                      tunnel: w418 -> [_ w450]
                      tunnel: w405 -> [_ w449]
                      frame False {
                      }
                      frame True {
                        n220 = call "获取最近两组水样测试数据.vi"("error in (no error)"=w450, "运行模式"=w449, "table"="pH") -> ("error out"=w454:errorcluster, "存储变量"=w453:T16)  [unwired: 7 in]
                        n221 = call "集成干预测试数据存储.vi"("error in (no error)"=w454, "存储变量"=w453) -> ("error out"=w451:errorcluster)  [unwired: 9 in]
                      }
                    }
                    n222 = global read "断电保存变量.vi" "DO"() -> (w410:bool)
                    n223 = case shown="真" w410 {
                      tunnel: [_ w445] -> w416
                      tunnel: w417 -> [_ w444]
                      tunnel: w405 -> [_ w443]
                      frame False {
                      }
                      frame True {
                        n224 = call "获取最近两组水样测试数据.vi"("error in (no error)"=w444, "运行模式"=w443, "table"="DO") -> ("error out"=w448:errorcluster, "存储变量"=w447:T16)  [unwired: 7 in]
                        n225 = call "集成干预测试数据存储.vi"("error in (no error)"=w448, "存储变量"=w447) -> ("error out"=w445:errorcluster)  [unwired: 9 in]
                      }
                    }
                    n226 = global read "断电保存变量.vi" "Cond"() -> (w409:bool)
                    n227 = case shown="真" w409 {
                      tunnel: [_ w439] -> w415
                      tunnel: w416 -> [_ w438]
                      tunnel: w405 -> [_ w437]
                      frame False {
                      }
                      frame True {
                        n228 = call "获取最近两组水样测试数据.vi"("error in (no error)"=w438, "运行模式"=w437, "table"="电导率") -> ("error out"=w442:errorcluster, "存储变量"=w441:T16)  [unwired: 7 in]
                        n229 = call "集成干预测试数据存储.vi"("error in (no error)"=w442, "存储变量"=w441) -> ("error out"=w439:errorcluster)  [unwired: 9 in]
                      }
                    }
                    n230 = global read "断电保存变量.vi" "Turb"() -> (w408:bool)
                    n231 = case shown="真" w408 {
                      tunnel: [_ w433] -> w414
                      tunnel: w415 -> [_ w432]
                      tunnel: w405 -> [_ w431]
                      frame False {
                      }
                      frame True {
                        n232 = call "获取最近两组水样测试数据.vi"("error in (no error)"=w432, "运行模式"=w431, "table"="浊度") -> ("error out"=w436:errorcluster, "存储变量"=w435:T16)  [unwired: 7 in]
                        n233 = call "集成干预测试数据存储.vi"("error in (no error)"=w436, "存储变量"=w435) -> ("error out"=w433:errorcluster)  [unwired: 9 in]
                      }
                    }
                    n234 = global read "断电保存变量.vi" "叶绿素a启用"() -> (w407:bool)
                    n235 = case shown="真" w407 {
                      tunnel: [_ w427] -> w413
                      tunnel: w414 -> [_ w426]
                      tunnel: w405 -> [_ w425]
                      frame False {
                      }
                      frame True {
                        n236 = call "获取最近两组水样测试数据.vi"("error in (no error)"=w426, "运行模式"=w425, "table"="叶绿素a") -> ("error out"=w430:errorcluster, "存储变量"=w429:T16)  [unwired: 7 in]
                        n237 = call "集成干预测试数据存储.vi"("error in (no error)"=w430, "存储变量"=w429) -> ("error out"=w427:errorcluster)  [unwired: 9 in]
                      }
                    }
                    n238 = global read "断电保存变量.vi" "藻密度"() -> (w406:bool)
                    n239 = case shown="真" w406 {
                      tunnel: [_ w421] -> _
                      tunnel: w413 -> [_ w420]
                      tunnel: w405 -> [_ w419]
                      frame False {
                      }
                      frame True {
                        n240 = call "获取最近两组水样测试数据.vi"("error in (no error)"=w420, "运行模式"=w419, "table"="藻密度") -> ("error out"=w424:errorcluster, "存储变量"=w423:T16)  [unwired: 7 in]
                        n241 = call "集成干预测试数据存储.vi"("error in (no error)"=w424, "存储变量"=w423) -> ("error out"=w421:errorcluster)  [unwired: 9 in]
                      }
                    }
                  }
                }
                n242 = case shown="真" w394 {
                  tunnel: w390 -> [_ w464]
                  frame False {
                  }
                  frame True {
                    n243 = call "获取最近两组水样测试数据.vi"("运行模式"=w464, "table"="CODMn") -> ("error out"=w465:errorcluster, "存储变量"=w466:T16)  [unwired: 8 in]
                    n244 = call "集成干预测试数据存储.vi"("error in (no error)"=w465, "存储变量"=w466) -> ()  [unwired: 9 in, 1 out]
                  }
                }
                n245 = case shown="真" w393 {
                  tunnel: w390 -> [_ w460]
                  frame False {
                  }
                  frame True {
                    n246 = call "获取最近两组水样测试数据.vi"("运行模式"=w460, "table"="CODCr") -> ("error out"=w461:errorcluster, "存储变量"=w462:T16)  [unwired: 8 in]
                    n247 = call "集成干预测试数据存储.vi"("error in (no error)"=w461, "存储变量"=w462) -> ()  [unwired: 9 in, 1 out]
                  }
                }
                n248 = case shown="真" w391 {
                  tunnel: w390 -> [_ w397]
                  frame False {
                  }
                  frame True {
                    n249 = call "获取最近两组水样测试数据.vi"("运行模式"=w397, "table"="总磷") -> ("error out"=w402:errorcluster, "存储变量"=w403:T16)  [unwired: 8 in]
                    n250 = call "集成干预测试数据存储.vi"("error in (no error)"=w402, "存储变量"=w403) -> ("error out"=w398:errorcluster)  [unwired: 9 in]
                    n251 = call "获取最近两组水样测试数据.vi"("error in (no error)"=w398, "运行模式"=w397, "table"="总氮") -> ("error out"=w401:errorcluster, "存储变量"=w400:T16)  [unwired: 7 in]
                    n252 = call "集成干预测试数据存储.vi"("error in (no error)"=w401, "存储变量"=w400) -> ()  [unwired: 9 in, 1 out]
                  }
                }
              }
            }
          }
        }
        n253 = global read "采配水全局变量.vi" "状态"() -> (w290:T9)
        n254 = Unbundle By Name(w290) -> ("R0"=w289:i16)
        n255 = Equal To 0?(x=w289) -> (x = 0?=w288:bool)
        n256 = Select(t=enum16{"初始化", "采配水启动", "仪器操作", "反冲洗", "结束"}."结束" ("枚举"), s=w288, f=enum16{"初始化", "采配水启动", "仪器操作", "反冲洗", "结束"}."反冲洗" ("枚举")) -> (s? t:f=w285:enum16{"初始化", "采配水启动", "仪器操作", "反冲洗", "结束"})
      }
      frame "结束" {
        n257 = Release Queue(queue=w476) -> ()  [unwired: 2 in, 3 out]
        n258 = Unbundle By Name(w473) -> ("测试模式"=w474:enum16{"正常测试", "集成干预"})
        n259 = Cancel Notification(0:w477) -> (8:w478:refnum<notifier>)  [unwired: 1 in, 2 out]
        n260 = Release Notifier(notifier=w478) -> ()  [unwired: 2 in, 3 out]
        n261 = case shown="\"集成干预\"" w474 {
          tunnel: w472 -> [_ w481]
          frame "正常测试", Default {
          }
          frame "集成干预" {
            n262 = global write "系统设置全局变量.vi" "运行模式"(w481) -> ()
          }
        }
      }
    }
    n263 = Format Into String(format string="%s,当前运行时间%d秒" ("格式字符串"), w15, w11) -> (resulting string=w16:string)  [unwired: 2 in, 1 out]
    n264 = global write "采配水全局变量.vi" "运行状态显示"(w16) -> ()
  }
